vi "F Dwf Analog In Channel Enable Set.vi"(8 "error in (no error)":errorcluster, 9 "fEnable":i32, 10 "idxChannel":i32, 11 "hdwf":i32) -> (0 "error out":errorcluster, 3 "function return":i32)   [LabVIEW 2024, in "Olasdwf.lvlib"]
doc: "DWFAPI int FDwfAnalogInChannelEnableSet(HDWF hdwf, int idxChannel, int fEnable);"
uses:
  Olasdwf.lvlib
  Windows/System32/dwf.dll
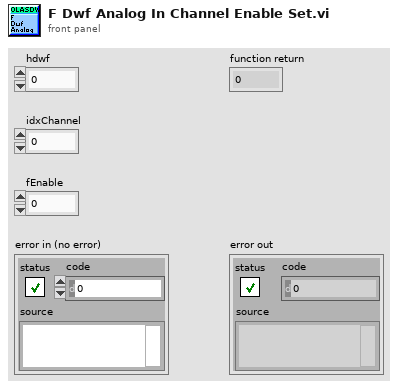
[diagram p1: front panel]
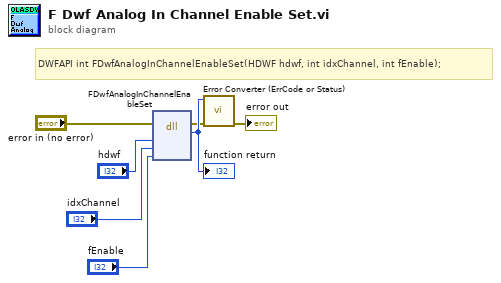
[diagram p0: block diagram]
diagram:
  # "DWFAPI int FDwfAnalogInChannelEnableSet(HDWF hdwf, int idxChannel, int fEnable);"
  n1 = dll-call lib="/Windows/System32/dwf.*" fn="FDwfAnalogInChannelEnableSet"(error in="error in (no error)", "hdwf"="hdwf", "idxChannel"="idxChannel", "fEnable"="fEnable") -> (error out=w2:errorcluster, w7:i32)  [unwired: 5 in, 1 out]
  "function return" <- w7
  n2 = call "Error Converter (ErrCode or Status).vi"("error in (no error)"=w2, "error code"=w7) -> ("error out"=→"error out":errorcluster)  [unwired: 9 in]
